vi "keyboardRemoteControl.vi"() -> ()   [LabVIEW 2020]
doc: "This example demonstrates how to read from a Play Station 4 controller using polling."
uses:
  <vilib>/Utility/inputDevices.llb/keyboardAcquire.vi
  <vilib>/Utility/inputDevices.llb/closeKeyboard.vi
  <vilib>/ReMiSYS Technology/RemoteToolkit/Sender/Sender.lvclass
panel:
  out "XY Speed":cluster{"X":i8, "Y":i8}
  in  "Stop Button":bool
  out "up":bool
  out "left":bool
  out "down":bool
  out "right":bool
  out "Y":i8(slide) scale=-100.0..100.0
  out "X":i8(slide) scale=-100.0..100.0
  out "XY Graph":cluster{i8[], i8[]}(graph)
  in  "IP Address":string="10.12.34.2"
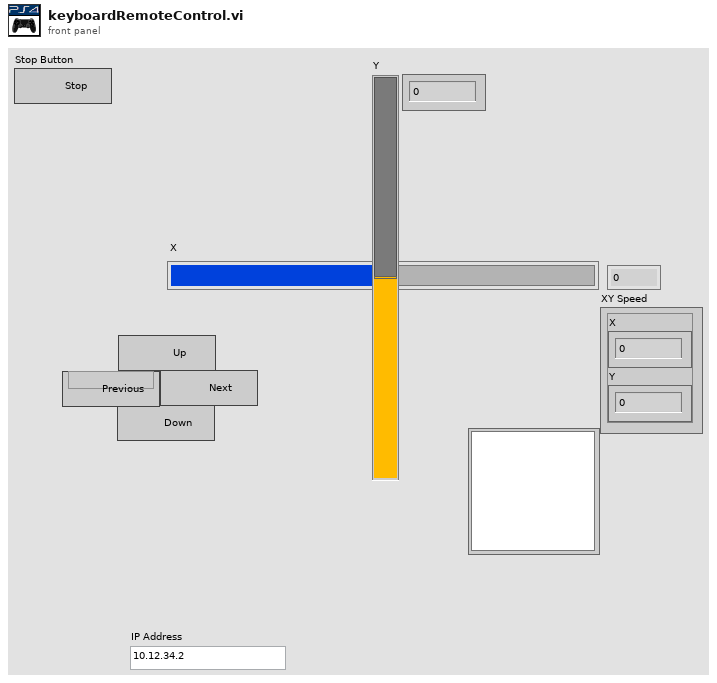
[diagram p1: front panel]
types:
  T1 = enum16{"0", "1", "2", "3", "4", "5", "6", "7", "8", "9", "A", "B", "C", "D", "E", "F", "G", "H", "I", "J", "K", "L", "M", "N", "O", "P", "Q", "R", "S", "T", "U", "V", "W", "X", "Y", "Z", "F1", "F2", "F3", "F4", "F5", "F6", "F7", "F8", "F9", "F10", "F11", "F12", "F13", "F14", "F15", "ADD", "BACK", "BACKSLASH", "CAPITAL", "COMMA", "DECIMAL", "DELETE", "DIVIDE", "DOWN", "END", "EQUALS", "ESCAPE", "GRAVE (`)", "HOME", "INSERT", "LBRACKET", "LCONTROL", "LEFT", "L ALT", "LSHIFT", "LWIN", "MINUS", "MULTIPLY", "NEXT", "NUMLOCK", "NUMPAD_0", "NUMPAD_1", "NUMPAD_2", "NUMPAD_3", "NUMPAD_4", "NUMPAD_5", "NUMPAD_6", "NUMPAD_7", "NUMPAD_8", "NUMPAD_9", "PAUSE", "PERIOD", "PRIOR (PG UP)", "RBRACKET", "RCONTROL", "RETURN", "RIGHT", "R ALT", "RSHIFT", "RWIN", "SCROLL", "SEMICOLON", "SLASH", "SPACE", "SUBTRACT", "TAB", "UP", "ENTER (num pad)", "' (quote)"}
  T2 = enum16{"0", "1", "2", "3", "4", "5", "6", "7", "8", "9", "A", "B", "C", "D", "E", "F", "G", "H", "I", "J", "K", "L", "M", "N", "O", "P", "Q", "R", "S", "T", "U", "V", "W", "X", "Y", "Z", "F1", "F2", "F3", "F4", "F5", "F6", "F7", "F8", "F9", "F10", "F11", "F12", "F13", "F14", "F15", "ADD", "BACK", "BACKSLASH", "CAPITAL", "COMMA", "DECIMAL", "DELETE", "DIVIDE", "DOWN", "END", "EQUALS", "ESCAPE", "GRAVE (`)", "HOME", "INSERT", "LBRACKET", "LCONTROL", "LEFT", "L ALT", "LSHIFT", "LWIN", "MINUS", "MULTIPLY", "NEXT", "NUMLOCK", "NUMPAD_0", "NUMPAD_1", "NUMPAD_2", "NUMPAD_3", "NUMPAD_4", "NUMPAD_5", "NUMPAD_6", "NUMPAD_7", "NUMPAD_8", "NUMPAD_9", "PAUSE", "PERIOD", "PRIOR (PG UP)", "RBRACKET", "RCONTROL", "RETURN", "RIGHT", "R ALT", "RSHIFT", "RWIN", "SCROLL", "SEMICOLON", "SLASH", "SPACE", "SUBTRACT", "TAB", "UP", "ENTER (num pad)", "' (quote)"}[]
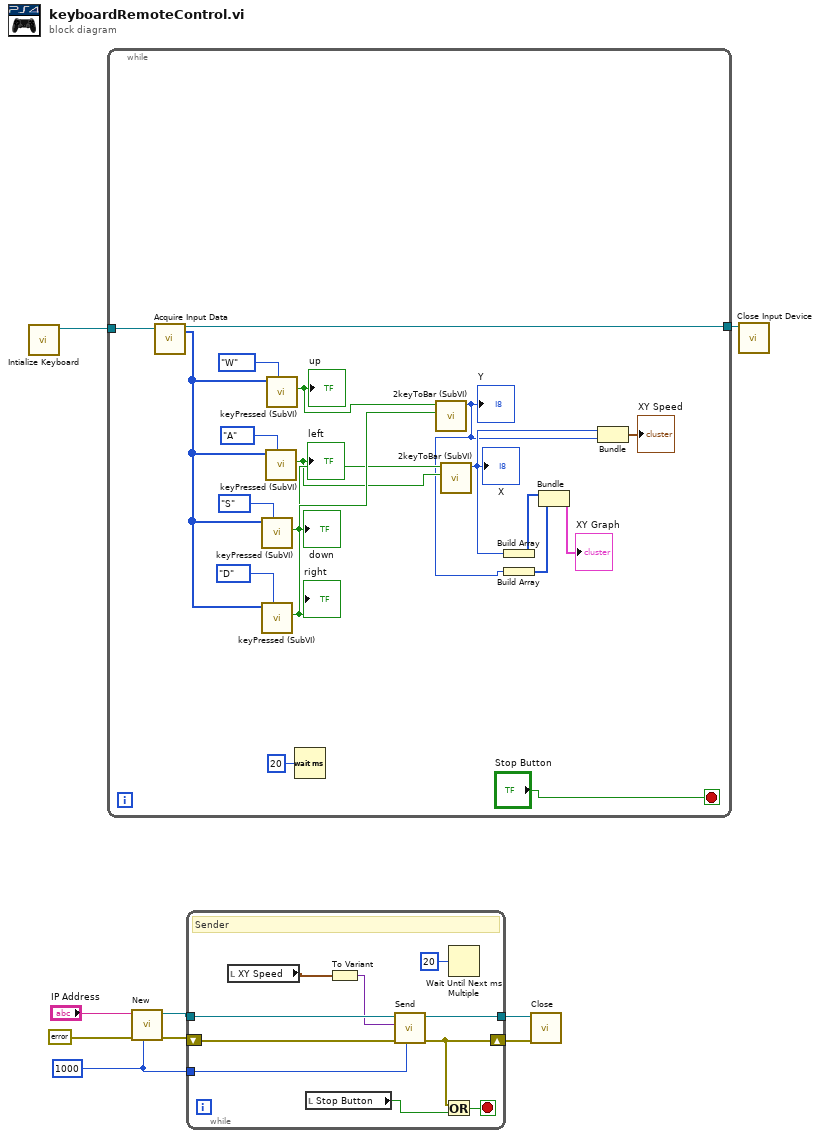
[diagram p0: block diagram]
diagram:
  w7 = 1000 ("Timeout ms (25000)")
  n1 = call <vilib>:"Intialize Keyboard.vi"() -> ("device ID"=w2:refnum<k1>)  [unwired: 10 in, 1 out]
  n2 = while {
    tunnel: w2 -> [w28]
    tunnel: [w27] -> w1
    stop <- "Stop Button" stop-if-true
    n3 = call-poly <vilib>:"Acquire Input Data.vi"("device ID"=w28) -> ("device ID"=w27:refnum<k1>, "keys pressed"=w21:T2)  [unwired: 16 in, 1 out]
    n4 = call "keyPressed (SubVI).vi"("keyNeeded"=T1."S", "keys pressed"=w21) -> ("keyPressed?"=w18:bool)  [unwired: 9 in]
    "down" <- w18
    n5 = call "keyPressed (SubVI).vi"("keyNeeded"=T1."D", "keys pressed"=w21) -> ("keyPressed?"=w17:bool)  [unwired: 9 in]
    "right" <- w17
    n6 = call "keyPressed (SubVI).vi"("keyNeeded"=T1."A", "keys pressed"=w21) -> ("keyPressed?"=w16:bool)  [unwired: 9 in]
    "left" <- w16
    n7 = call "keyPressed (SubVI).vi"("keyNeeded"=T1."W", "keys pressed"=w21) -> ("keyPressed?"=w20:bool)  [unwired: 9 in]
    "up" <- w20
    n8 = Wait (ms)(milliseconds to wait=u32 20) -> ()  [unwired: 1 out]
    n9 = call "2keyToBar (SubVI).vi"("NegKey"=w18, "PosKey"=w20) -> ("Output"=w11:i8)  [unwired: 9 in]
    "Y" <- w11
    n10 = call "2keyToBar (SubVI).vi"("NegKey"=w16, "PosKey"=w17) -> ("Output"=w12:i8)  [unwired: 9 in]
    "X" <- w12
    n11 = Build Array(w12) -> (w15:i8[])
    n12 = Build Array(w11) -> (w14:i8[])
    n13 = Bundle(w15, w14) -> (→"XY Graph":cluster{i8[], i8[]})  [unwired: 1 in]
    n14 = Bundle("Output"=w12, "Output"=w11) -> (→"XY Speed":cluster{"Output":i8, "Output":i8})  [unwired: 1 in]
  }
  n15 = call <vilib>:"New.vi"("Timeout ms (25000)"=w7, "Error In"=errorcluster {"status"=FALSE, "code"=0, "source"=""}, "IP Address"="IP Address") -> ("Error Out"=w8:errorcluster, "Sender Ref."=w5:refnum<class "Sender.lvclass">)  [unwired: 7 in]
  n16 = while {
    shift-right: [w34] -> w4
    shift-left: w8 -> [w36]
    tunnel: w5 -> [w37]
    tunnel: w7 -> [w32]
    tunnel: [w35] -> w3
    stop <- w38 stop-if-true
    # "Sender"
    n17 = local read "XY Speed"() -> (w30:cluster{"X":i8, "Y":i8})
    n18 = local read "Stop Button"() -> (w29:bool)
    n19 = To Variant(anything=w30) -> (Variant=w33:variant)
    n20 = call <vilib>:"Send.vi"("Timeout ms (1000)"=w32, "Error In"=w36, "Value"=w33, "Sender Ref."=w37) -> ("Error Out"=w34:errorcluster, "Sender Ref."=w35:refnum<class "Sender.lvclass">)  [unwired: 6 in]
    n21 = Or(x=w34, y=w29) -> (x .or. y?=w38:bool)
    n22 = Wait Until Next ms Multiple(millisecond multiple=u32 20) -> ()  [unwired: 1 out]
  }
  n23 = call <vilib>:"Close.vi"("Error In"=w4, "Receiver Ref."=w3) -> ()  [unwired: 9 in, 1 out]
  n24 = call-poly <vilib>:"Close Input Device.vi"("device ID"=w1) -> ()  [unwired: 9 in, 1 out]
